vi "Read Configuration (Template).vi"   [LabVIEW 2019, in "Configuration.lvclass"]
uses:
  Configuration.lvclass
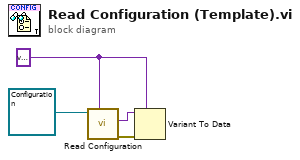
[diagram p0: block diagram]
diagram:
  w1 = variant ("INI Fomatted Cluster Type")
  n1 = call "Read Configuration.vi"("INI Fomatted Cluster Type"=w1, "Configuration in"=refnum<class "Configuration.lvclass"> refnum) -> ("error out"=w3:errorcluster, "Configuration"=w4:variant)  [unwired: 7 in, 1 out]
  n2 = Variant To Data(error in=w3, type=w1, Variant=w4) -> ()  [unwired: 2 out]
